vi "UTIL_OPEN and LOAD QUEUE for Reentrant v1_0_0.vi"(6 "Queue elements":string[](array[string])=["Initialize"], 7 "Flush queue first":bool, 8 "error in (no error)":errorcluster, 11 "Call Chain":string[](array[string])) -> (0 "error out":errorcluster, 3 "Queue out":refnum<queue>)   [LabVIEW 2009]
doc: "UTIL_OPEN and LOAD QUEUE for Re-entrant v1_0_0.vi\n\nCreates/Loads a queue by the name of the calling vi (minus the extension.vi) then a : and the clone Id. It then either flushes the items already on the queue then adds any additional Queue elements or just simply adds any new Queue elements to the queue and passes the queue reference out.\n\nCreated 2006 by\n\nJ. Daren Suntych\nNational Analytics\n970-397-0764"
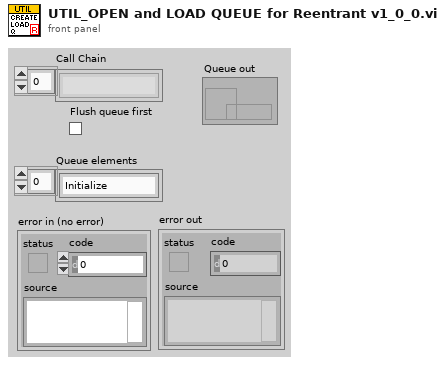
[diagram p1: front panel]
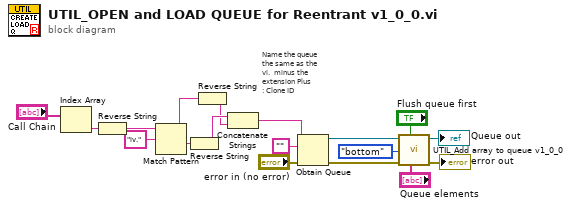
[diagram p0: block diagram]
diagram:
  # "Name the queue\nthe same as the\nvi.  minus the\nextension Plus\n: Clone ID"
  n1 = Index Array(array="Call Chain") -> (element=w5:string)  [unwired: 1 in]
  n2 = Reverse String(1:w5) -> (0:w7:string)
  n3 = Match Pattern(string=w7, regular expression="iv.") -> (before substring=w4:string, after substring=w8:string)  [unwired: 3 out]
  n4 = Reverse String(1:w8) -> (0:w3:string)
  n5 = Reverse String(1:w4) -> (0:w2:string)
  n6 = Concatenate Strings(w3, w2) -> (w1:string)
  n7 = Obtain Queue(name (unnamed)=w1, element data type="", error in (no error)="error in (no error)") -> (queue out=w16:refnum<queue>, error out=w15:errorcluster)  [unwired: 2 in, 1 out]
  n8 = call "UTIL_Add array to queue v1_0_0.vi"("Queue elements"="Queue elements", "Flush (f)"="Flush queue first", "error in (no error)"=w15, "Queue position"=enum16{"top", "bottom"}."bottom", "Queue in"=w16) -> ("error out"=→"error out":errorcluster, "Queue out"=→"Queue out":refnum<queue>)  [unwired: 5 out]
